vi "stop.vi"() -> ()   [LabVIEW 2018]
panel:
  in  "?":bool
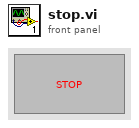
[diagram p1: front panel]
types:
  T1 = typedef "LVPositionTypeDef.ctl" = cluster{"Left":i32, "Top":i32}
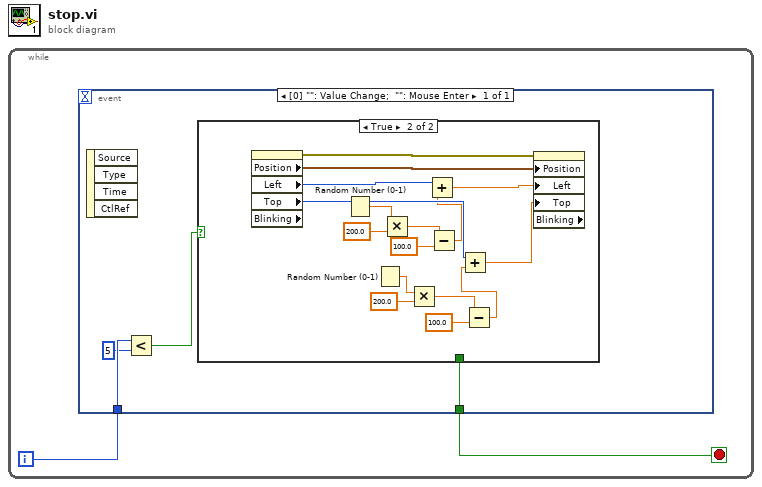
[diagram p0: block diagram]
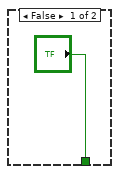
[diagram p2: hidden frame]
diagram:
  n1 = while {
    i -> [w2]
    stop <- w1 stop-if-true
    n2 = event shown="[0] \"\": Value Change;  \"\": Mouse Enter" {
      selector: _ -> [_]
      dyn-events: _ -> [_]
      timeout: _ -> [_]
      tunnel: w2 -> [w5]
      tunnel: [w6] -> w1
      event Value Change; Mouse Enter {
        n3 = event-data() -> ()  [unwired: 1 in, 4 out]
        n4 = Less?(x=w5, y=5) -> (x < y?=w3:bool)
        n5 = case shown="True" w3 {
          tunnel: ["?" _] -> w6
          frame False {
          }
          frame True {
            n6 = property class="Bool" props=["Position", "Left", "Top", "Blinking"]() -> (error out=w23:errorcluster, "Position"=w22:T1, "Left"=w19:i32, "Top"=w17:i32)  [unwired: 2 in, 2 out]
            n7 = Random Number (0-1)() -> (number: 0 to 1=w21:dbl)
            n8 = Random Number (0-1)() -> (number: 0 to 1=w16:dbl)
            n9 = Multiply(x=w21, y=200.0) -> (x*y=w13:dbl)
            n10 = Multiply(x=w16, y=200.0) -> (x*y=w10:dbl)
            n11 = Subtract(x=w13, y=100.0) -> (x-y=w11:dbl)
            n12 = Add(x=w19, y=w11) -> (x+y=w18:dbl)
            n13 = Subtract(x=w10, y=100.0) -> (x-y=w8:dbl)
            n14 = Add(x=w17, y=w8) -> (x+y=w14:dbl)
            n15 = property class="Bool" props=["Position", "Left", "Top", "Blinking"](error in=w23, "Position"=w22, "Left"=w18, "Top"=w14) -> ()  [unwired: 1 in, 3 out]
          }
        }
      }
    }
  }
